vi "Request Element by Name.vi"(8 "error in (no error)":errorcluster, 10 "Name":string, 11 "Look Up Table in":refnum<class "Look Up Table.lvclass">) -> (0 "error out":errorcluster, 1 "Found?":bool, 2 "Element":variant, 3 "Look Up Table out":refnum<class "Look Up Table.lvclass">)   [LabVIEW 2016, in "Stream Look Up Table.lvlib" / "Look Up Table.lvclass"]
doc: "--\nCopyright © 2017 Composed SystemsI All rights reserved.\n\nAuthor: Jon McBee <jon.mcbee@composed.io>\n\nThis library is provided \"AS IS\" ,WITHOUT WARRANTIES OR\nCONDITIONS OF ANY KIND, either express or implied.\n\nComposed Systems -- composed.io\n\nStream 0.0.1.1\nJon McBee - Composed Systems\nCopyright (c) 2017, Composed Systems"
uses:
  <userlib>/Composed Systems/Stream/Look Up Table/Look Up Table/Look Up Table.lvclass
  <userlib>/Composed Systems/Stream/Look Up Table/Look Up Table/Look Up Table.lvclass/Look Up Table.ctl
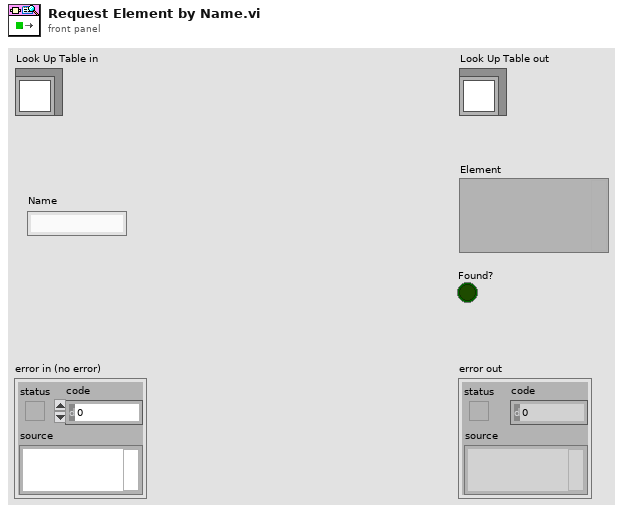
[diagram p1: front panel]
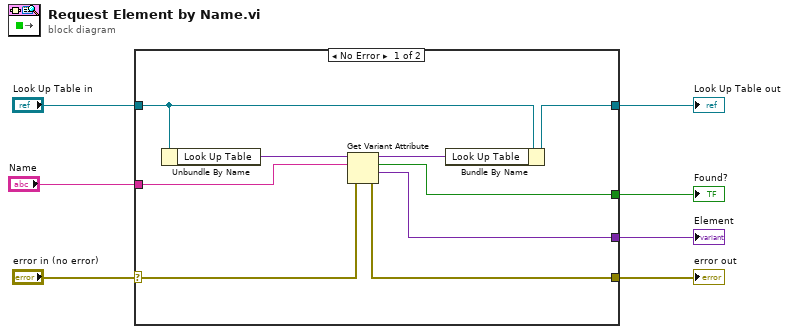
[diagram p0: block diagram]
diagram:
  n1 = case shown="No Error" "error in (no error)" {
    selector: "error in (no error)" -> [w12 w18]
    tunnel: [w11 w18] -> w6
    tunnel: [w15 w17] -> w4
    tunnel: "Look Up Table in" -> [w16 w17]
    tunnel: "Name" -> [w13 _]
    tunnel: [w8 _] -> w2
    tunnel: [w10 _] -> w1
    frame No Error {
      n2 = Unbundle By Name(w16) -> ("Look Up Table"=w14:variant)
      n3 = Get Variant Attribute(Variant=w14, name=w13, error in=w12) -> (duplicate Variant=w9:variant, found=w10:bool, value=w8:variant, error out=w11:errorcluster)  [unwired: 1 in]
      n4 = Bundle By Name(cluster=w16, "Look Up Table"=w9) -> (w15:refnum<class "Look Up Table.lvclass">)
    }
    frame Error {
    }
  }
  "error out" <- w6
  "Look Up Table out" <- w4
  "Found?" <- w1
  "Element" <- w2
